vi "initializer_load_spec.vi"(9 "LUA Specification File":path, 10 "Parameters Tree":refnum<vi>, 11 "# Lines":refnum<vi>) -> (2 "Spec File Loaded":bool)   [LabVIEW 2019]
uses:
  lib/libSimulationControl/libSimulationControl.lvlib
  lib/libSpecValiReader/libSpecValiReader.lvlib
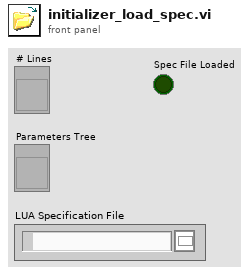
[diagram p1: front panel]
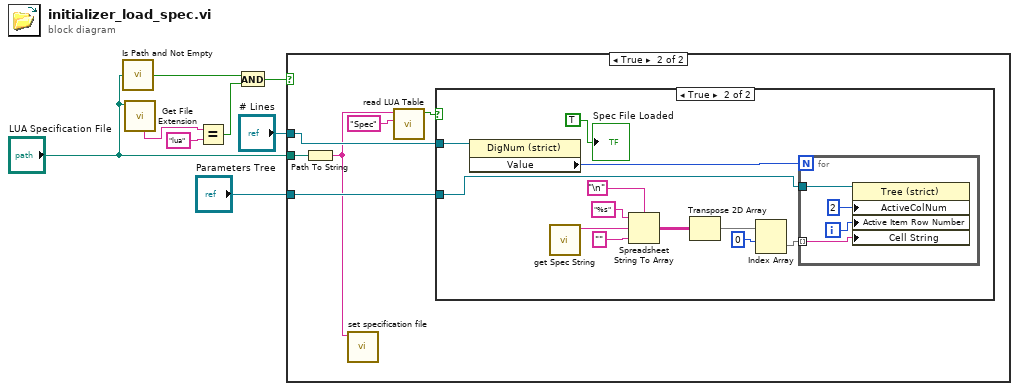
[diagram p0: block diagram]
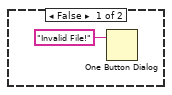
[diagram p2: hidden frame]
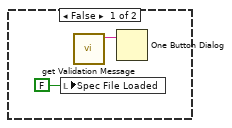
[diagram p3: hidden frame]
diagram:
  n1 = call <vilib>:"Is Path and Not Empty.vi"("path"="LUA Specification File") -> ("Is Path and Not Empty?"=w4:bool)  [unwired: 4 in]
  n2 = call <vilib>:"Get File Extension.vi"("file"="LUA Specification File") -> ("unmodified file extension"=w6:string)  [unwired: 6 in, 4 out]
  n3 = Equal?(x=w6, y="lua") -> (x = y?=w3:bool)
  n4 = And(x=w4, y=w3) -> (x .and. y?=w1:bool)
  n5 = case shown="True" w1 {
    tunnel: "Parameters Tree" -> [_ w15]
    tunnel: "# Lines" -> [_ w14]
    tunnel: "LUA Specification File" -> [_ w13]
    frame False {
      n6 = One Button Dialog(message="Invalid File!") -> ()  [unwired: 1 in, 1 out]
    }
    frame True {
      n7 = Path To String(path=w13) -> (string=w10:string)
      n8 = call "set specification file.vi"("spec_file"=w10) -> ()  [unwired: 10 in, 1 out]
      n9 = call "read LUA Table.vi"("vali_or_spec"="Spec" ("spec_filename"), "filename"=w10) -> ("function return"=w12:bool)  [unwired: 8 in, 1 out]
      n10 = case shown="True" w12 {
        tunnel: w15 -> [_ w28]
        tunnel: w14 -> [_ w27]
        frame False {
          n11 = local write "Spec File Loaded"(FALSE ("Spec File Loaded")) -> ()
          n12 = call "get Validation Message.vi"() -> ("function return"=w16:string)  [unwired: 10 in, 1 out]
          n13 = One Button Dialog(message=w16) -> ()  [unwired: 1 in, 1 out]
        }
        frame True {
          n14 = property class="DigNum (strict)"(reference=w27) -> ("Value"=w20:i32)  [unwired: 1 in, 2 out]
          n15 = call "get Spec String.vi"() -> ("function return"=w18:string)  [unwired: 10 in, 1 out]
          n16 = Spreadsheet String To Array(delimiter (Tab)="\n", format string="%s", spreadsheet string=w18, array type (2D Dbl)="") -> (array=w25:string[][])
          n17 = Transpose 2D Array(2D array=w25) -> (transposed array=w26:string[][])
          n18 = Index Array(array=w26, index (row)=0) -> (element=w29:string[])  [unwired: 1 in]
          n19 = for {
            N: w20 -> [_]
            tunnel: w29 -> [w31] mode=indexing
            tunnel: w28 -> [w30]
            i -> [w32]
            n20 = property on="Property Node" class="Tree (strict)"(reference=w30, "ActiveColNum"=2 ("Active Cell:Active Column Number"), "Active Item Row Number"=w32, "Cell String"=w31) -> ()  [unwired: 1 in, 2 out]
          }
          "Spec File Loaded" <- TRUE ("Value")
        }
      }
    }
  }
